vi "Calculate Color Index Array.vi"(8 "error in (no error)":errorcluster, 10 "3D Waterfall Datatype in":refnum<class "3D Waterfall Datatype.lvclass">, 11 "Plot Representation In":T1) -> (0 "error out":errorcluster, 2 "3D Waterfall Datatype out":refnum<class "3D Waterfall Datatype.lvclass">, 3 "Plot Representation Out":T1)   [LabVIEW 2017, in "3D Waterfall Datatype.lvclass"]
uses:
  <vilib>/Math Plots/3D Math Plots/3D Waterfall/3D Waterfall Datatype/3D Waterfall Datatype.lvclass
  <vilib>/Math Plots/3D Math Plots/3D Plot/3D Plot/Typedef/Plot Representation.ctl
  <vilib>/Math Plots/3D Math Plots/3D Plot/3D Plot/Typedef/Range Clusters.ctl
  <vilib>/Math Plots/3D Math Plots/3D Plot/3D Plot/Typedef/Mesh Data.ctl
  <vilib>/Math Plots/3D Math Plots/3D Waterfall/3D Waterfall Datatype/3D Waterfall Datatype.lvclass/3D Waterfall Datatype.ctl
  <vilib>/Math Plots/3D Math Plots/3D Plot/3D Plot Datatype/3D Plot Datatype.lvclass
  <vilib>/Math Plots/3D Math Plots/3D Plot/3D Plot/3D Plot.lvclass
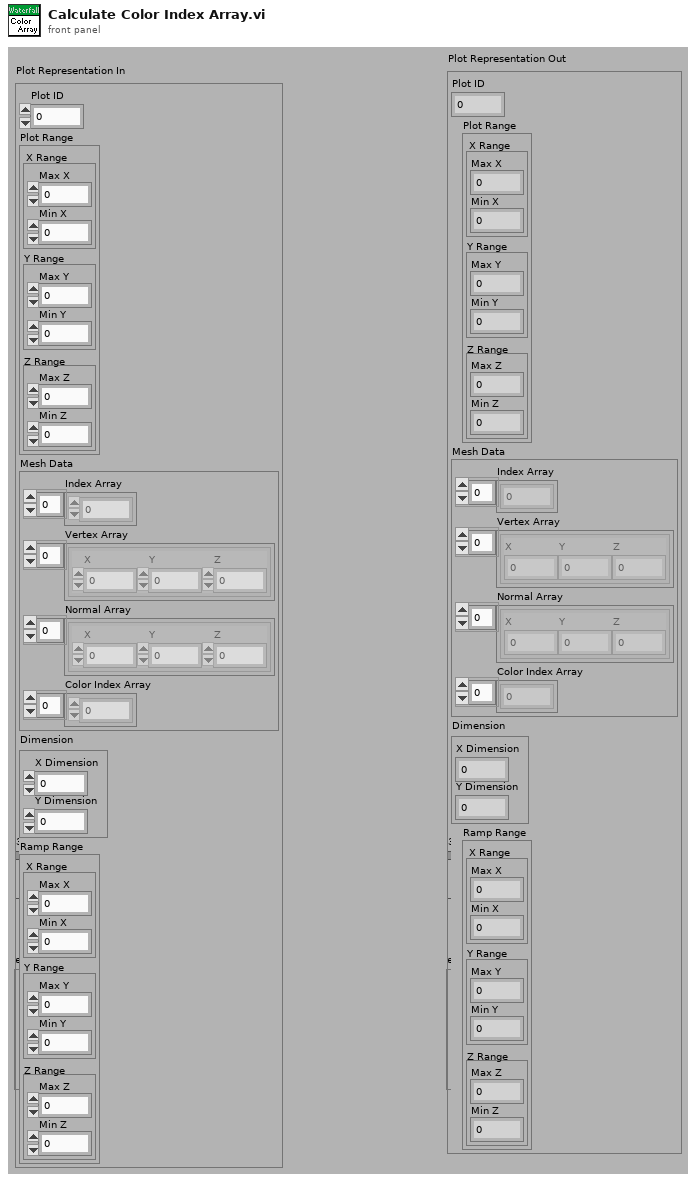
[diagram p1: front panel]
types:
  T1 = typedef "3D Plot.lvclass/Plot Representation.ctl" = cluster{"Plot ID":i32, "Plot Range":T2, "Mesh Data":T3, "Dimension":cluster{"X Dimension":i32, "Y Dimension":i32}, "Ramp Range":T2}
  T2 = typedef "3D Plot.lvclass/Range Clusters.ctl" = cluster{"X Range":cluster{"Max X":sgl, "Min X":sgl}, "Y Range":cluster{"Max Y":sgl, "Min Y":sgl}, "Z Range":cluster{"Max Z":sgl, "Min Z":sgl}}
  T3 = typedef "3D Plot.lvclass/Mesh Data.ctl" = cluster{"Index Array":u32[], "Vertex Array":cluster{"X":sgl, "Y":sgl, "Z":sgl}[], "Normal Array":cluster{"X":sgl, "Y":sgl, "Z":sgl}[], "Color Index Array":i32[]}
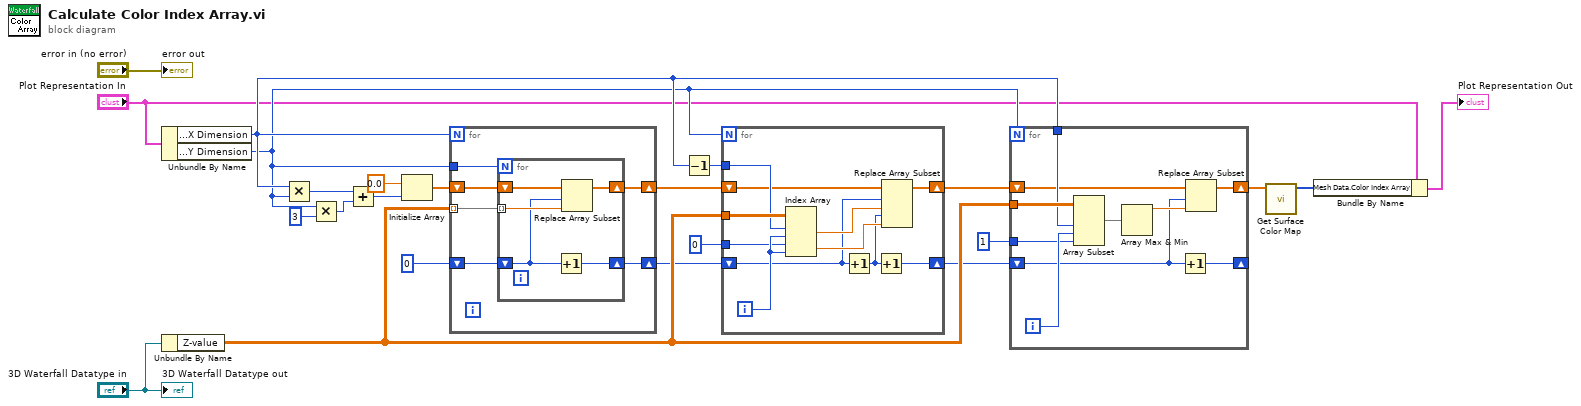
[diagram p0: block diagram]
diagram:
  n1 = Unbundle By Name("Plot Representation In") -> ("Dimension.X Dimension"=w15:i32, "Dimension.Y Dimension"=w12:i32)
  n2 = Unbundle By Name("3D Waterfall Datatype in") -> ("Z-value"=w14:sgl[][])
  n3 = Multiply(x=w15, y=w12) -> (x*y=w7:i32)
  n4 = Multiply(x=w12, y=3 ("x")) -> (x*y=w6:i32)
  n5 = Add(x=w7, y=w6) -> (x+y=w5:i32)
  n6 = Initialize Array(sgl 0.0 ("element"), w5) -> (w19:sgl[])
  n7 = for {
    N: w15 -> [_]
    tunnel: w12 -> [w29]
    shift-right: [w24] -> w11
    shift-left: w19 -> [w28]
    tunnel: w14 -> [w27] mode=indexing
    shift-right: [w26] -> w10
    shift-left: 0 -> [w25]
    n8 = for {
      N: w29 -> [_]
      shift-right: [w33] -> w24
      shift-left: w28 -> [w34]
      tunnel: w27 -> [w32] mode=indexing
      shift-right: [w31] -> w26
      shift-left: w25 -> [w30]
      n9 = Increment(x=w30) -> (x+1=w31:i32)
      n10 = Replace Array Subset(array=w34, new element=w32, index=w30) -> (w33:sgl[])
    }
  }
  n11 = Decrement(x=w15) -> (x-1=w16:i32)
  n12 = for {
    N: w12 -> [_]
    shift-right: [w40] -> w9
    shift-left: w11 -> [w41]
    tunnel: w14 -> [w45]
    tunnel: w16 -> [w44]
    tunnel: 0 -> [w42]
    shift-right: [w37] -> w8
    shift-left: w10 -> [w35]
    i -> [w43]
    n13 = Index Array(array=w45, index (row) #1=w44, index (col) #1=w43, index (row) #2=w42, index (col) #2=w43) -> (element #1=w39:sgl, element #2=w38:sgl)
    n14 = Increment(x=w35) -> (x+1=w36:i32)
    n15 = Increment(x=w36) -> (x+1=w37:i32)
    n16 = Replace Array Subset(array=w41, new element #1=w39, index #1=w35, new element #2=w38, index #2=w36) -> (w40:sgl[])
  }
  n17 = for {
    N: w12 -> [_]
    tunnel: w14 -> [w55]
    tunnel: w15 -> [w52]
    shift-right: [w50] -> w2
    shift-left: w9 -> [w51]
    shift-right: [w48] -> _
    shift-left: w8 -> [w47]
    tunnel: 1 ("length") -> [w46]
    i -> [w53]
    n18 = Array Subset(array=w55, length (row)=w52, index (col)=w53, length (col)=w46) -> (w54:sgl[][])  [unwired: 1 in]
    n19 = Array Max & Min(array=w54) -> (max value=w49:sgl)  [unwired: 3 out]
    n20 = Increment(x=w47) -> (x+1=w48:i32)
    n21 = Replace Array Subset(array=w51, new element=w49, index=w47) -> (w50:sgl[])
  }
  n22 = call <vilib>:"Get Surface Color Map.vi"("Amplifiy"=w2) -> ("Color Index Array"=w21:i32[])  [unwired: 1 in, 9 out]
  n23 = Bundle By Name(cluster="Plot Representation In", "Mesh Data.Color Index Array"=w21) -> (→"Plot Representation Out":T1)
  "error out" <- "error in (no error)"
  "3D Waterfall Datatype out" <- "3D Waterfall Datatype in"
